vi "Teststand Post Sub Steps Template.vi"(11 "Sequence Context In":refnum<k7>) -> (0 "error out":errorcluster, 3 "Report Text":string)   [LabVIEW 2023, in "LTT_TeststandSteptypes.lvlib"]
uses:
  LTT_TeststandSteptypes.lvlib
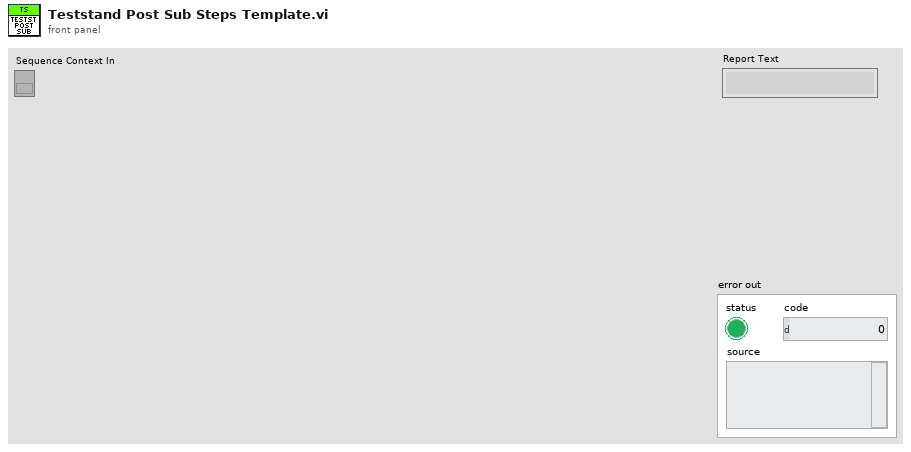
[diagram p1: front panel]
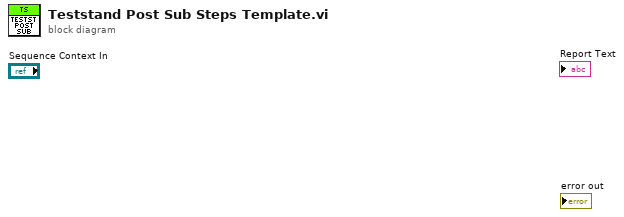
[diagram p0: block diagram]
diagram:
